vi "LS336_Temp_Readout_DP_ver2.0.vi"(0 "GPIB ADR (18)":i16=18, 1 "Enable ChD (F)":bool=TRUE, 7 "Mode: (default: 2)":i16(ring)=2 items=["Do nothing to mark the end of the transfer", "Send NL (linefeed) with EOI after the data bytes.", "Send EOI with the last data byte in the string(default)"], 11 "error in":errorcluster) -> (2 "Sensor A (K)":dbl format="%.3f", 3 "Sensor A (K)":string, 4 "dump GPIB ADR":i16, 6 "Sensor B (K)":dbl format="%.3f", 8 "Sensor B (K)":string, 10 "Sensor C (K)":dbl format="%.3f", 12 "Sensor D (K)":dbl format="%.3f", 13 "Sensor D (K)":string, 14 "error out":errorcluster, 15 "Sensor C (K)":string)   [LabVIEW 2012]
doc: "This returns the field in the sample chamber as reported by the PPMS system. Note that this is not the exact field, only that calculated from the current through the magnet."
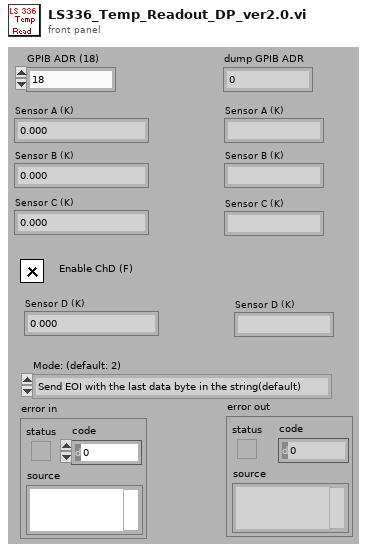
[diagram p1: front panel]
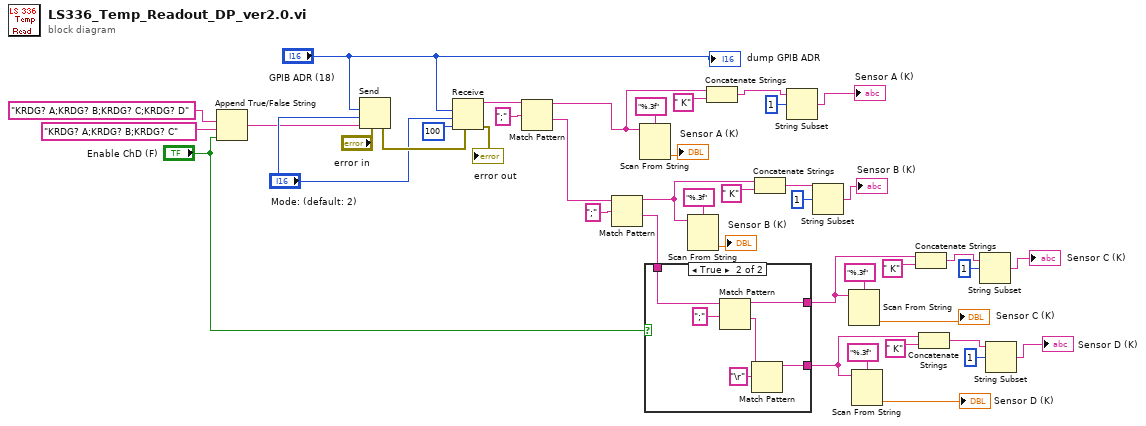
[diagram p0: block diagram]
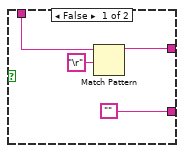
[diagram p2: hidden frame]
diagram:
  n1 = Append True/False String(1:"Enable ChD (F)", 2:"KRDG? A;KRDG? B;KRDG? C", 3:"KRDG? A;KRDG? B;KRDG? C;KRDG? D") -> (0:w20:string)  [unwired: 1 out]
  n2 = Send(2:"GPIB ADR (18)", 3:"Mode: (default: 2)", 4:"error in", 5:w20) -> (8:w34:errorcluster)  [unwired: 1 in, 2 out]
  n3 = Receive(4:w34, 6:100, 7:"Mode: (default: 2)", 8:"GPIB ADR (18)") -> (0:→"error out":errorcluster, 3:w36:string)  [unwired: 1 in, 2 out]
  n4 = Match Pattern(string=w36, regular expression=";") -> (before substring=w32:string, after substring=w30:string)  [unwired: 3 out]
  n5 = Match Pattern(string=w30, regular expression=";") -> (before substring=w26:string, after substring=w16:string)  [unwired: 3 out]
  n6 = Scan From String(format string="%.3f", input string=w32) -> (output 1=→"Sensor A (K)":dbl)  [unwired: 2 in, 4 out]
  n7 = case shown="True" "Enable ChD (F)" {
    tunnel: w16 -> [w45 w52]
    tunnel: [w46 w49] -> w14
    tunnel: ["" w48] -> w13
    frame False {
      n8 = Match Pattern(string=w45, regular expression="\r") -> (before substring=w46:string)  [unwired: 4 out]
    }
    frame True {
      n9 = Match Pattern(string=w52, regular expression=";") -> (before substring=w49:string, after substring=w51:string)  [unwired: 3 out]
      n10 = Match Pattern(string=w51, regular expression="\r") -> (before substring=w48:string)  [unwired: 4 out]
    }
  }
  n11 = Scan From String(format string="%.3f", input string=w26) -> (output 1=→"Sensor B (K)":dbl)  [unwired: 2 in, 4 out]
  n12 = Concatenate Strings(w32, " K" ("string")) -> (w7:string)
  n13 = Concatenate Strings(w26, " K" ("string")) -> (w5:string)
  n14 = String Subset(string=w7, offset (0)=1) -> (substring=→"Sensor A (K)":string)  [unwired: 1 in]
  n15 = String Subset(string=w5, offset (0)=1) -> (substring=→"Sensor B (K)":string)  [unwired: 1 in]
  n16 = Scan From String(format string="%.3f", input string=w14) -> (output 1=→"Sensor C (K)":dbl)  [unwired: 2 in, 4 out]
  n17 = Scan From String(format string="%.3f", input string=w13) -> (output 1=→"Sensor D (K)":dbl)  [unwired: 2 in, 4 out]
  n18 = Concatenate Strings(w14, " K" ("string")) -> (w4:string)
  n19 = Concatenate Strings(w13, " K" ("string")) -> (w2:string)
  n20 = String Subset(string=w4, offset (0)=1) -> (substring=→"Sensor C (K)":string)  [unwired: 1 in]
  n21 = String Subset(string=w2, offset (0)=1) -> (substring=→"Sensor D (K)":string)  [unwired: 1 in]
  "dump GPIB ADR" <- "GPIB ADR (18)"
